vi "ROSmsg_IsArray.vi"(11 "type in":string) -> (0 "array size":i32, 2 "Is Array?":bool, 3 "type out":string)   [LabVIEW 2015]
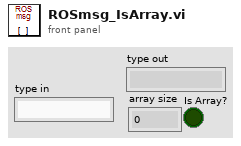
[diagram p1: front panel]
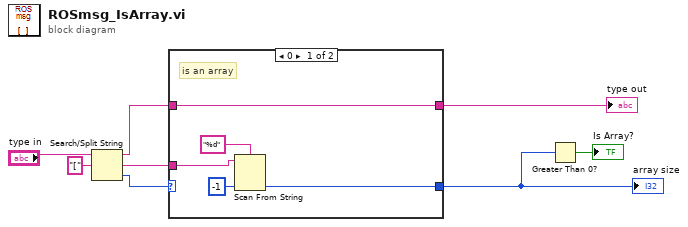
[diagram p0: block diagram]
diagram:
  n1 = Search/Split String(string="type in", search string/char (-)="[") -> (substring before match=w8:string, match + rest of string=w7:string, offset of match=w6:i32)  [unwired: 1 in]
  n2 = case shown="0" w6 {
    selector: w6 -> [_ w14]
    tunnel: w7 -> [w13 _]
    tunnel: w8 -> [w10 w15]
    tunnel: [w10 w15] -> w3
    tunnel: [w9 w14] -> w2
    frame 0 {
      # "is an array"
      n3 = Scan From String(format string="%d", input string=w13, default 1=-1 ("default value 1")) -> (output 1=w9:i32)  [unwired: 2 in, 3 out]
    }
    frame -1, Default {
      # "not an array"
    }
  }
  "type out" <- w3
  "array size" <- w2
  n4 = Greater Than 0?(x=w2) -> (x > 0?=→"Is Array?":bool)
